vi "SPI Read Write.vi"(0 "handle":u32 format="%08x", 1 "outBuffer":string, 11 "error in (no error)":errorcluster, 13 "transferOptions":u32=6 format="%x") -> (4 "handle out":u32 format="%08x", 6 "sizeTransferred":u32, 8 "inBuffer":string, 15 "error out":errorcluster)   [LabVIEW 2018, in "libMPSSE-SPI.lvlib"]
doc: "FTDI_API FT_STATUS SPI_ReadWrite(FT_HANDLE handle, uint8 *inBuffer,\n uint8 *outBuffer, uint32 sizeToTransfer, uint32 *sizeTransferred,\n uint32 transferOptions);"
uses:
  libMPSSE-SPI.lvlib
  dll/libMPSSE.dll
panel:
  # "/* transferOptions-Bit0: If this bit is 0 then it means that the transfer size provided is in bytes */\n#define\tSPI_TRANSFER_OPTIONS_SIZE_IN_BYTES\t\t\t0x00000000\n/* transferOptions-Bit0: If this bit is 1 then it means that the transfer size provided is in bytes */\n#define\tSPI_TRANSFER_OPTIONS_SIZE_IN_BITS\t\t\t0x00000001\n/* transferOptions-Bit1: if BIT1 is 1 then CHIP_SELECT line will be enabled at start of transfer */\n#define\tSPI_TRANSFER_OPTIONS_CHIPSELECT_ENABLE\t\t0x00000002\n/* transferOptions-Bit2: if BIT2 is 1 then CHIP_SELECT line will be disabled at end of transfer */\n#define SPI_TRANSFER_OPTIONS_CHIPSELECT_DISABLE\t\t0x00000004"
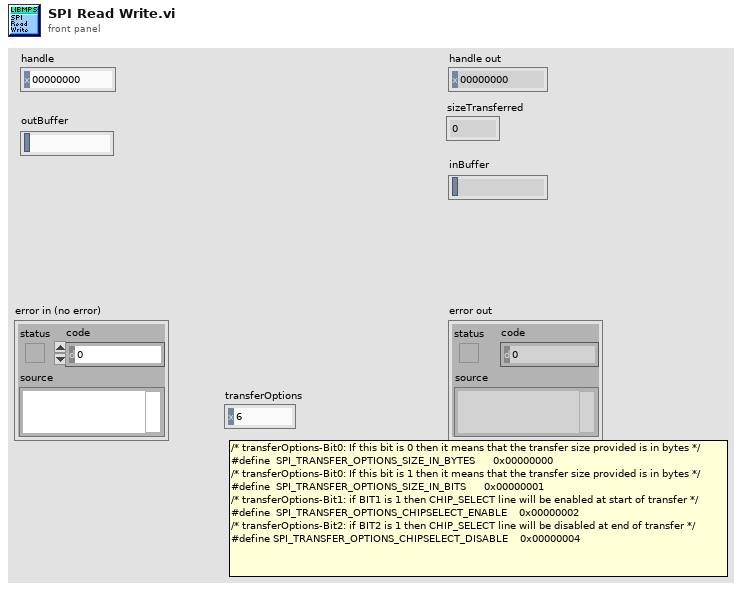
[diagram p1: front panel]
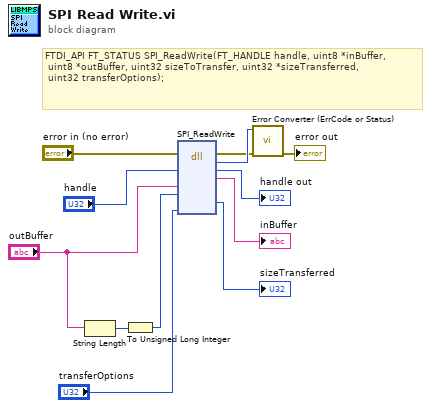
[diagram p0: block diagram]
diagram:
  # "FTDI_API FT_STATUS SPI_ReadWrite(FT_HANDLE handle, uint8 *inBuffer,\n\tuint8 *outBuffer, uint32 sizeToTransfer, uint32 *sizeTransferred,\n\tuint32 transferOptions);"
  n1 = String Length(string="outBuffer") -> (length=w4:i32)
  n2 = To Unsigned Long Integer(number=w4) -> (unsigned 32bit integer=w3:u32)
  n3 = dll-call lib="D:/LABVIEW/Examples - 32bit/FTDI/libMPSSE-SPI-LabVIEW-master/dll/libMPSSE.*" fn="SPI_ReadWrite"(error in="error in (no error)", "handle"="handle", "outBuffer"="outBuffer", "sizeToTransfer"=w3, "transferOptions"="transferOptions") -> (error out=w6:errorcluster, "return type"=w12:u32, "handle"=→"handle out":u32, "inBuffer"=→"inBuffer":string, "sizeTransferred"=→"sizeTransferred":u32)  [unwired: 7 in, 1 out]
  n4 = call "Error Converter (ErrCode or Status).vi"("error in (no error)"=w6, "error code"=w12) -> ("error out"=→"error out":errorcluster)  [unwired: 9 in]
